vi "氨氮总磷质控流程.vi"(0 "队列输入":refnum<queue>, 5 "氨氮":bool, 7 "氨氮量程切换":enum32{"H", "L", "AUTO"}(ring)=enum."AUTO", 9 "总磷":bool, 11 "总磷量程切换":enum32{"H", "L", "AUTO"}(ring)=enum."AUTO") -> (4 "布尔":bool, 6 "总磷中断报警":bool, 8 "氨氮中断报警":bool)   [LabVIEW 2016, in "质控单元.lvlib"]
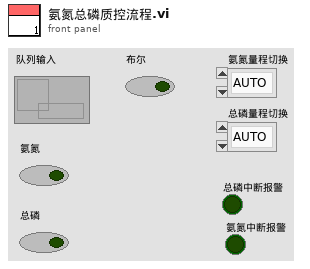
[diagram p1: front panel]
types:
  T1 = enum16{"待机", "启动氨氮水样", "氨氮测量中", "启动氨氮加标", "启动氨氮加标回收", "氨氮加标回收测量中", "启动总磷水样", "总磷水样测量中", "启动总磷加标", "启动总磷加标回收", "总磷加标回收测量中", "结束"}
  T2 = cluster{"站号":u16, "量程切换":enum32{"H", "L", "AUTO"}, "控制命令":enum16{"启动测量", "标样核查", "零点核查", "跨度核查", "空白测试", "平行样测试", "加标回收", "空白校准", "标样校准", "初始化（清洗）", "停止测试", "仪器重启", "校时", "模式设置", "测量间隔设置", "盲样测试"}, "模式设置":enum16{"待机", "连续模式", "周期模式", "定点模式", "受控模式", "手动模式"}, "测量间隔":u16}
  T3 = cluster{"时间标识":timestamp, "设备":string, "日志信息":string}
  T4 = cluster{"系统时间":timestamp, "工作状态":enum16{"空闲", "水样测试", "标样核查", "零点核查", "跨度核查", "空白测试", "平行样测试", "加标回收", "空白校准", "标样校准", "初始化（清洗）"}, "测量模式":enum16{"待机", "连续模式", "周期模式", "定点模式", "受控模式", "手动模式"}, "告警代码":enum16{"无告警", "缺试剂告警", "缺水样告警", "缺蒸馏水告警", "缺标液告警", "仪表漏液告警", "标定异常告警", "超量程告警", "加热异常", "低试剂预警", "超上限告警", "超下限告警", "仪表内部其他异常", "滴定异常告警", "电极异常告警", "量程切换告警", "参数设置告警", "PH电极电位异常", "电导率电极异常", "浊度光度异常", "溶解氧电极异常", "溶解氧光强异常", "温度异常告警", "PH异常告警", "溶解氧异常告警", "电导率异常告警", "浊度异常告警", "叶绿素异常告警", "藻密度异常告警", "蓝绿藻异常告警", "ORP异常告警", "氨氮异常告警", "清洁刷异常告警", "SD卡异常告警", "蓝牙异常告警", "Wifi异常告警", "流程异常告警"}, "故障代码":enum16{"无故障", "电机故障", "温度故障", "通讯故障", "滴定故障"}, "日志代码":u16, "软件版本":u16, "F0":sgl, "F1":sgl, "F2":sgl, "F3":sgl, "T":sgl, "H":sgl, "id":u16, "flowid":u16, "量程":u16, "总磷控温温度1":sgl, "营养盐控温温度2":sgl, "ADC":sgl}
  T5 = enum16{"空闲", "水样测试", "标样核查", "零点核查", "跨度核查", "空白测试", "平行样测试", "加标回收", "空白校准", "标样校准", "初始化（清洗）"}
  T6 = cluster{"因子编码":u32, "单位":u16, "标样参考值":sgl, "水样数据时间":timestamp, "水样实测值":sgl, "水样数据标识":string, "标样数据时间":timestamp, "标样实测值":sgl, "标样数据标识":string, "空白数据时间":timestamp, "空白实测值":sgl, "空白数据标识":string, "零点核查数据时间":timestamp, "零点核查实测值":sgl, "零点核查数据标识":string, "跨度核查数据时间":timestamp, "跨度核查实测值":sgl, "跨度核查数据标识":string, "加标回收数据时间":timestamp, "加标回收实测值":sgl, "加标回收数据标识":string, "平行样数据时间":timestamp, "平行样实测值":sgl, "平行样数据标识":string}
  T7 = cluster{"量程":dbl, "检出限":dbl, "加标前水样浓度":dbl, "加标后水样浓度":dbl, "加标水杯定容体积":dbl, "加标母液浓度":dbl, "加标体积":dbl, "加标回收率":dbl}
  T8 = cluster{"氨氮":u8, "总磷":u8, "总氮":u8, "CODMn":u8, "CODCr":u8}
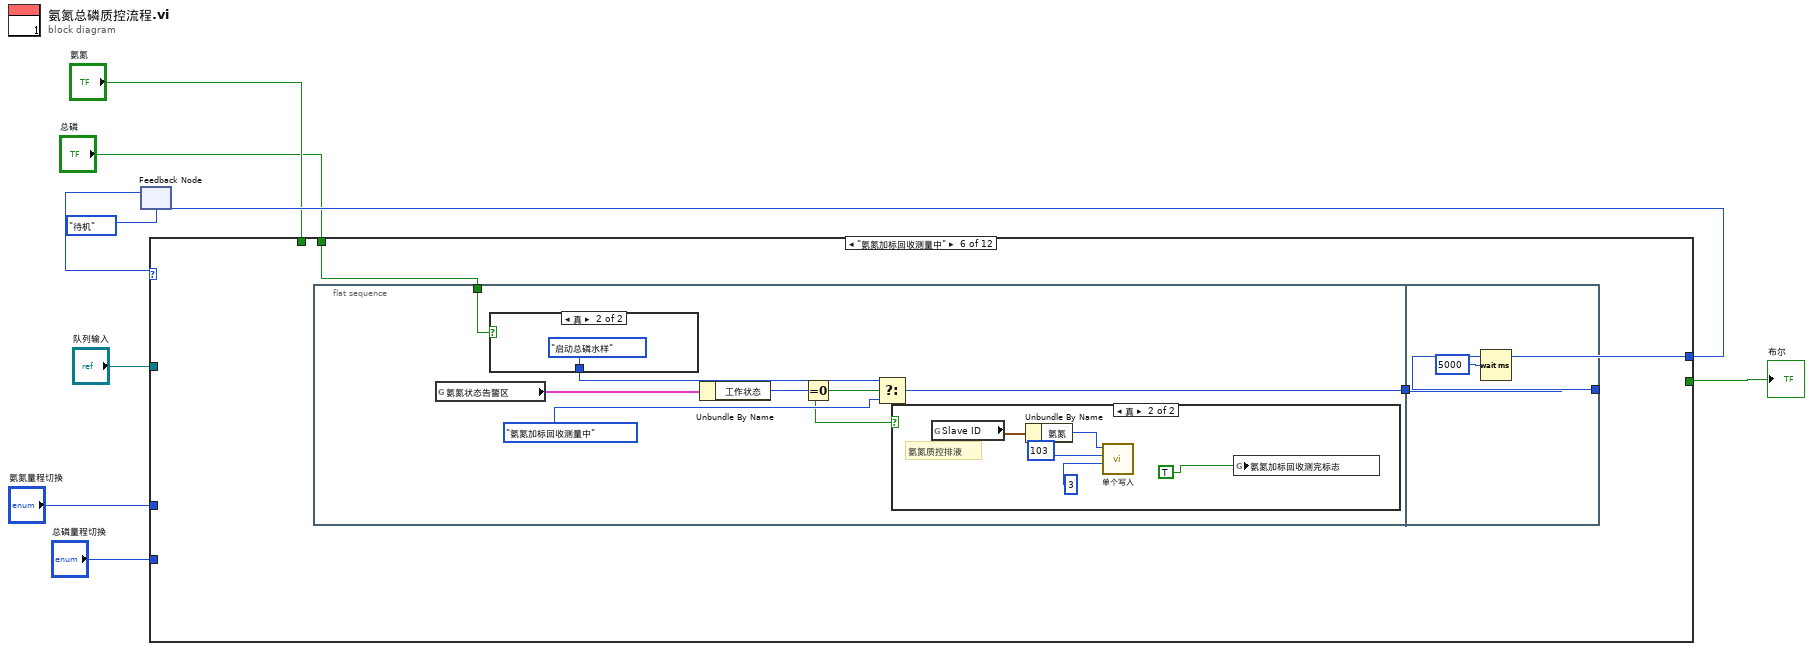
[diagram p0: block diagram]
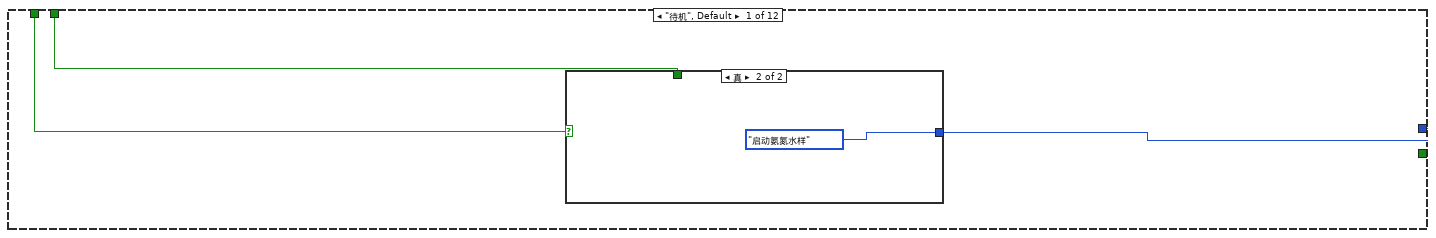
[diagram p2: hidden frame]
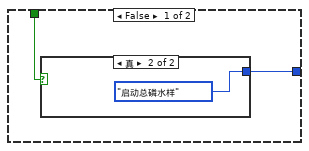
[diagram p3: hidden frame]
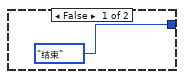
[diagram p4: hidden frame]
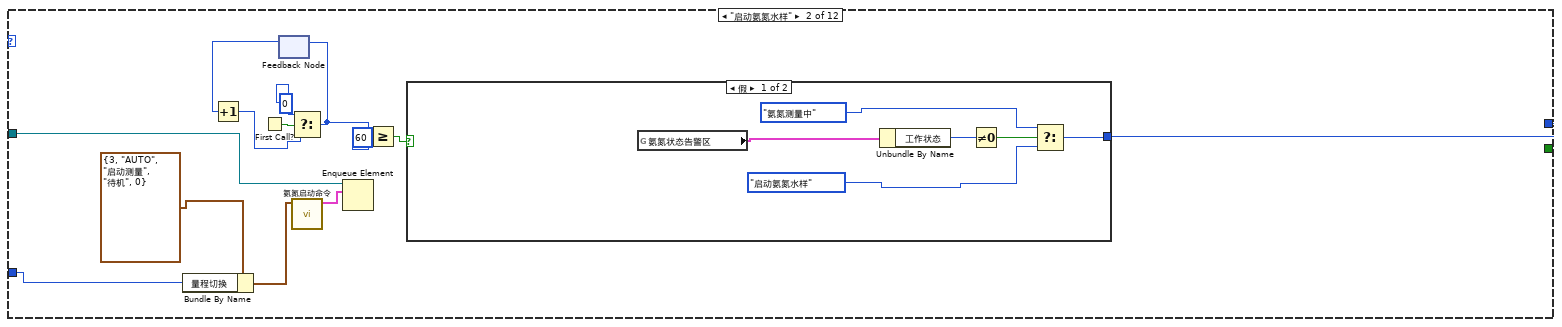
[diagram p5: hidden frame]
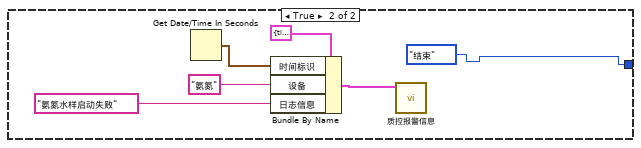
[diagram p6: hidden frame]
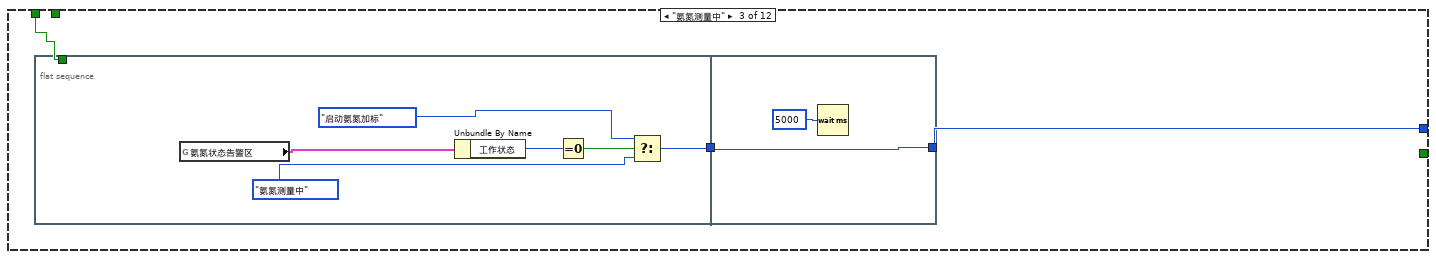
[diagram p7: hidden frame]
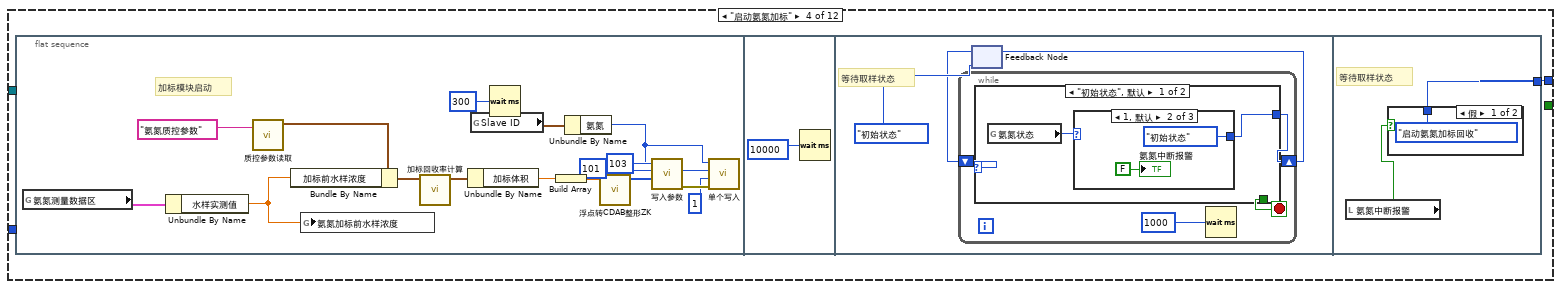
[diagram p8: hidden frame]
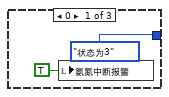
[diagram p9: hidden frame]
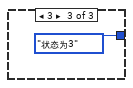
[diagram p10: hidden frame]
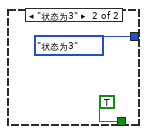
[diagram p11: hidden frame]
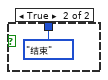
[diagram p12: hidden frame]
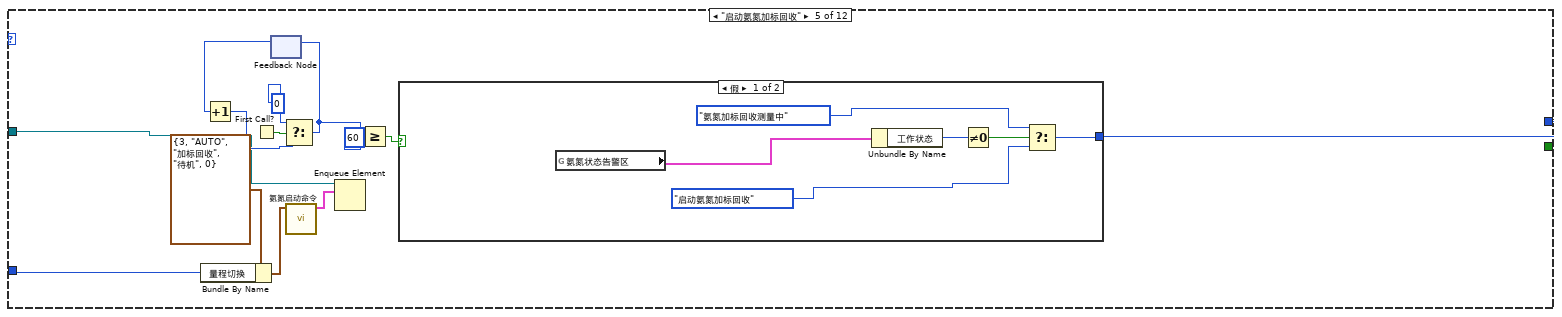
[diagram p13: hidden frame]
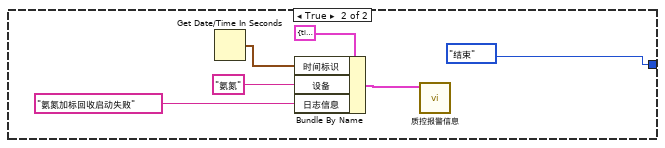
[diagram p14: hidden frame]
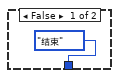
[diagram p15: hidden frame]
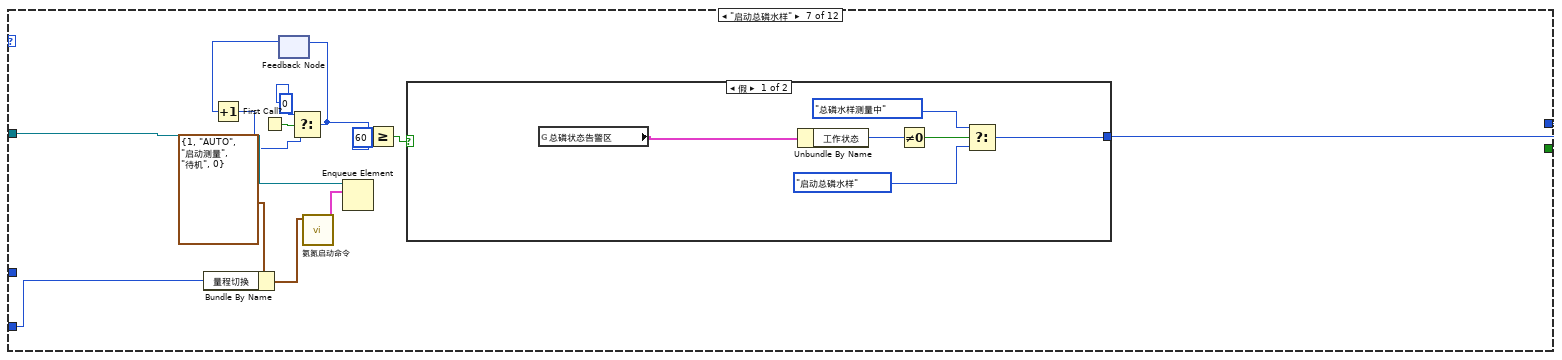
[diagram p17: hidden frame]
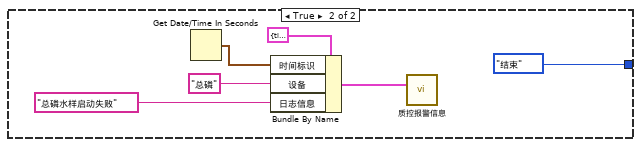
[diagram p18: hidden frame]
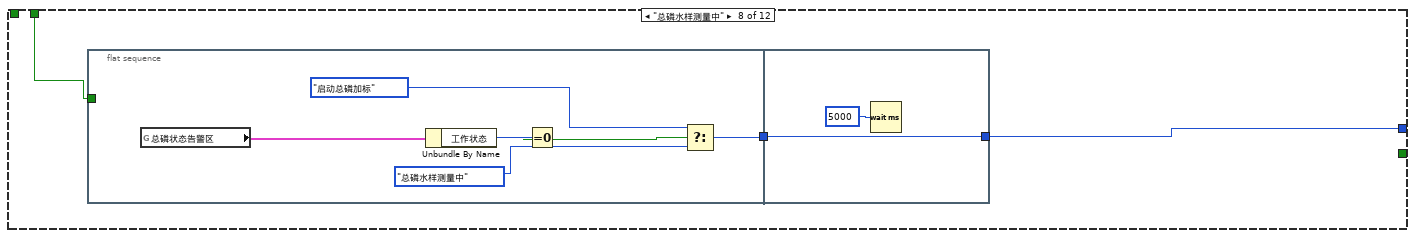
[diagram p19: hidden frame]
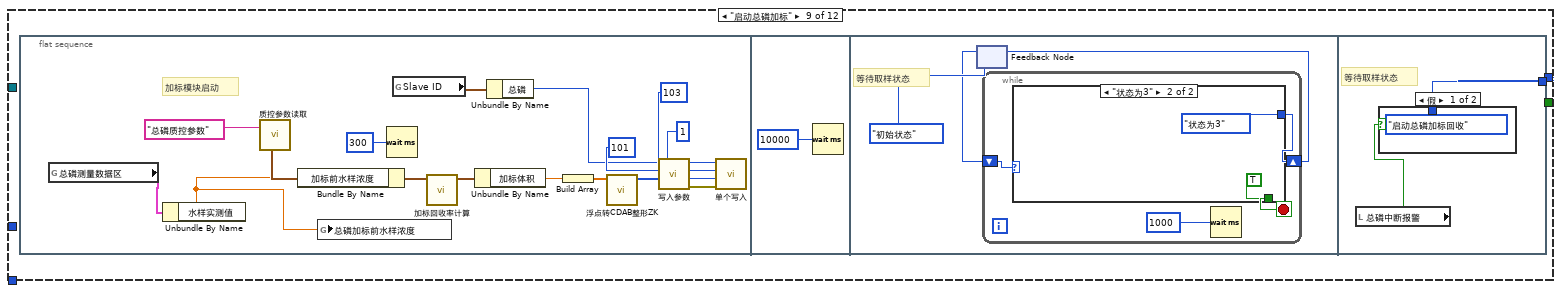
[diagram p20: hidden frame]
diagram:
  n1 = feedback #1(T1."待机") -> (w8:T1)
  n2 = case shown="\"氨氮加标回收测量中\"" w8 {
    tunnel: [w12 w29 w45 w54 w96 w118 w147 w163 w172 w214 w235 T1."结束"] -> w7
    tunnel: "队列输入" -> [_ w30 _ _ w97 _ w148 _ _ w215 _ _]
    tunnel: [_ _ _ _ _ _ _ _ _ _ _ TRUE] -> w4
    tunnel: "总磷" -> [w10 _ _ _ _ w117 _ w161 _ _ _ _]
    tunnel: "氨氮" -> [w11 _ w43 _ _ _ _ _ _ _ _ _]
    tunnel: "氨氮量程切换" -> [_ w19 _ _ w93 _ _ _ _ _ _ _]
    tunnel: "总磷量程切换" -> [_ _ _ _ _ _ w136 _ _ w213 _ _]
    frame "待机", Default {
      n3 = case shown="真" w11 {
        tunnel: [w13 T1."启动氨氮水样"] -> w12
        tunnel: w10 -> [w14 _]
        frame False {
          n4 = case shown="真" w14 {
            tunnel: [T1."结束" T1."启动总磷水样"] -> w13
            frame False {
            }
            frame True {
            }
          }
        }
        frame True {
        }
      }
    }
    frame "启动氨氮水样" {
      n5 = Bundle By Name(cluster=T2 {"站号"=3, "量程切换"=enum."AUTO", "控制命令"=enum."启动测量", "模式设置"=enum."待机", "测量间隔"=0} ("参数"), "量程切换"=w19) -> (w18:T2)
      n6 = First Call?() -> (First Call?: T/F=w27:bool)
      n7 = feedback #2() -> (w26:i32)  [unwired: 1 in]
      n8 = Increment(x=w26) -> (x+1=w25:i32)
      n9 = Select(t=0, s=w27, f=w25) -> (s? t:f=w24:i32)
      n10 = feedback-in #2(w24) -> ()
      n11 = call "氨氮启动命令.vi"("参数"=w18) -> ("启动命令"=w21:cluster{"命令":string, "data":variant})  [unwired: 10 in]
      n12 = Enqueue Element(queue=w30, element=w21) -> ()  [unwired: 2 in, 3 out]
      n13 = Greater Or Equal?(x=w24, y=60) -> (x >= y?=w22:bool)
      n14 = case shown="假" w22 {
        tunnel: [w34 T1."结束"] -> w29
        frame False {
          n15 = global read "与氨氮交互全局.vi" "氨氮状态告警区"() -> (w31:T4)
          n16 = Unbundle By Name(w31) -> ("工作状态"=w36:T5)
          n17 = Not Equal To 0?(x=w36) -> (x != 0?=w35:bool)
          n18 = Select(t=T1."氨氮测量中", s=w35, f=T1."启动氨氮水样") -> (s? t:f=w34:T1)
        }
        frame True {
          n19 = Get Date/Time In Seconds() -> (seconds since 1Jan1904=w42:timestamp)
          n20 = Bundle By Name(cluster=T3 {"时间标识"=timestamp(0 s since 1904-01-01), "设备"="", "日志信息"=""} ("data in"), "时间标识"=w42, "设备"="氨氮", "日志信息"="氨氮水样启动失败") -> (w38:T3)
          n21 = call "质控报警信息.vi"("data in"=w38) -> ()  [unwired: 11 in]
        }
      }
    }
    frame "氨氮测量中" {
      n22 = flat-sequence {
        tunnel: [w50] -> w44
        tunnel: w43 -> [_]
        tunnel: [w53] -> w45
        tunnel: w44 -> [w53]
        frame #0 {
          n23 = global read "与氨氮交互全局.vi" "氨氮状态告警区"() -> (w46:T4)
          n24 = Unbundle By Name(w46) -> ("工作状态"=w51:T5)
          n25 = Equal To 0?(x=w51) -> (x = 0?=w49:bool)
          n26 = Select(t=T1."启动氨氮加标", s=w49, f=T1."氨氮测量中") -> (s? t:f=w50:T1)
        }
        frame #1 {
          n27 = Wait (ms)(milliseconds to wait=u32 5000 ("等待时间（毫秒）")) -> ()  [unwired: 1 out]
        }
      }
    }
    frame "启动氨氮加标" {
      n28 = flat-sequence {
        tunnel: [w89] -> w54
        frame #0 {
          # "加标模块启动"
          n29 = global read "与氨氮交互全局.vi" "氨氮测量数据区"() -> (w58:T6)
          n30 = Unbundle By Name(w58) -> ("水样实测值"=w59:sgl)
          n31 = call "质控参数读取.vi"("section"="氨氮质控参数") -> ("参数"=w68:T7)  [unwired: 9 in, 1 out]
          n32 = Bundle By Name(cluster=w68, "加标前水样浓度"=w59) -> (w69:T7)
          n33 = global write "水样浓度全局.vi" "氨氮加标前水样浓度"(w59) -> ()
          n34 = call "加标回收率计算.vi"("参数"=w69) -> ("参数 out"=w67:T7)  [unwired: 9 in, 1 out]
          n35 = Unbundle By Name(w67) -> ("加标体积"=w60:dbl)
          n36 = global read "断电保存全局.vi" "Slave ID"() -> (w56:T8)
          n37 = Wait (ms)(milliseconds to wait=u32 300 ("等待时间（毫秒）")) -> ()  [unwired: 1 out]
          n38 = Build Array(w60) -> (w66:dbl[])
          n39 = Unbundle By Name(w56) -> ("氨氮"=w55:u8)
          n40 = call "浮点转CDAB整形ZK.vi"("浮点数"=w66) -> ("CDAB整形输出"=w61:u16[])  [unwired: 10 in]
          n41 = call "写入参数.vi"("values"=w61, "starting address"=u16 101, "Slave ID"=w55) -> ("error out"=w65:errorcluster)  [unwired: 8 in]
          n42 = call "单个写入.vi"("Error in"=w65, "value"=u16 1, "address"=u16 103, "Slave ID"=w55) -> ()  [unwired: 7 in, 1 out]
        }
        frame #1 {
          n43 = Wait (ms)(milliseconds to wait=u32 10000 ("等待时间（毫秒）")) -> ()  [unwired: 1 out]
        }
        frame #2 {
          # "等待取样状态"
          n44 = feedback #3(enum16{"初始状态", "状态为3"}."初始状态") -> (w73:enum16{"初始状态", "状态为3"})
          n45 = while {
            shift-right: [w77] -> w72
            shift-left: w73 -> [w78]
            stop <- w76 stop-if-true
            n46 = case shown="\"初始状态\", 默认" w78 {
              tunnel: [w80 enum16{"初始状态", "状态为3"}."状态为3"] -> w77
              tunnel: [_ TRUE] -> w76
              frame "初始状态", Default {
                n47 = global read "加标回收状态全局变量.vi" "氨氮状态"() -> (w79:u16)
                n48 = case shown="1, 默认" w79 {
                  tunnel: [enum16{"初始状态", "状态为3"}."状态为3" enum16{"初始状态", "状态为3"}."初始状态" enum16{"初始状态", "状态为3"}."状态为3"] -> w80
                  frame 0 {
                    n49 = local write "氨氮中断报警"(TRUE ("氨氮中断报警")) -> ()
                  }
                  frame 1, Default {
                    "氨氮中断报警" <- FALSE ("氨氮中断报警")
                  }
                  frame 3 {
                  }
                }
              }
              frame "状态为3" {
              }
            }
            n50 = Wait (ms)(milliseconds to wait=u32 1000 ("等待时间（毫秒）")) -> ()  [unwired: 1 out]
          }
          n51 = feedback-in #3(w72) -> ()
        }
        frame #3 {
          # "等待取样状态"
          n52 = local read "氨氮中断报警"() -> (w88:bool)
          n53 = case shown="假" w88 {
            tunnel: [T1."启动氨氮加标回收" T1."结束"] -> w89
            frame False {
            }
            frame True {
            }
          }
        }
      }
    }
    frame "启动氨氮加标回收" {
      n54 = Bundle By Name(cluster=T2 {"站号"=3, "量程切换"=enum."AUTO", "控制命令"=enum."加标回收", "模式设置"=enum."待机", "测量间隔"=0} ("参数"), "量程切换"=w93) -> (w92:T2)
      n55 = First Call?() -> (First Call?: T/F=w103:bool)
      n56 = feedback #4() -> (w102:i32)  [unwired: 1 in]
      n57 = Increment(x=w102) -> (x+1=w101:i32)
      n58 = Select(t=0, s=w103, f=w101) -> (s? t:f=w100:i32)
      n59 = feedback-in #4(w100) -> ()
      n60 = call "氨氮启动命令.vi"("参数"=w92) -> ("启动命令"=w95:cluster{"命令":string, "data":variant})  [unwired: 10 in]
      n61 = Enqueue Element(queue=w97, element=w95) -> ()  [unwired: 2 in, 3 out]
      n62 = Greater Or Equal?(x=w100, y=60) -> (x >= y?=w98:bool)
      n63 = case shown="假" w98 {
        tunnel: [w108 T1."结束"] -> w96
        frame False {
          n64 = global read "与氨氮交互全局.vi" "氨氮状态告警区"() -> (w105:T4)
          n65 = Unbundle By Name(w105) -> ("工作状态"=w110:T5)
          n66 = Not Equal To 0?(x=w110) -> (x != 0?=w109:bool)
          n67 = Select(t=T1."氨氮加标回收测量中", s=w109, f=T1."启动氨氮加标回收") -> (s? t:f=w108:T1)
        }
        frame True {
          n68 = Get Date/Time In Seconds() -> (seconds since 1Jan1904=w116:timestamp)
          n69 = Bundle By Name(cluster=T3 {"时间标识"=timestamp(0 s since 1904-01-01), "设备"="", "日志信息"=""} ("data in"), "时间标识"=w116, "设备"="氨氮", "日志信息"="氨氮加标回收启动失败") -> (w112:T3)
          n70 = call "质控报警信息.vi"("data in"=w112) -> ()  [unwired: 11 in]
        }
      }
    }
    frame "氨氮加标回收测量中" {
      n71 = flat-sequence {
        tunnel: [w125] -> w119
        tunnel: w117 -> [w121]
        tunnel: [w135] -> w118
        tunnel: w119 -> [w135]
        frame #0 {
          n72 = global read "与氨氮交互全局.vi" "氨氮状态告警区"() -> (w120:T4)
          n73 = case shown="真" w121 {
            tunnel: [T1."结束" T1."启动总磷水样"] -> w123
            frame False {
            }
            frame True {
            }
          }
          n74 = Unbundle By Name(w120) -> ("工作状态"=w126:T5)
          n75 = Equal To 0?(x=w126) -> (x = 0?=w122:bool)
          n76 = Select(t=w123, s=w122, f=T1."氨氮加标回收测量中") -> (s? t:f=w125:T1)
          n77 = case shown="真" w122 {
            frame False {
            }
            frame True {
              # "氨氮质控排液"
              n78 = global read "断电保存全局.vi" "Slave ID"() -> (w130:T8)
              n79 = Unbundle By Name(w130) -> ("氨氮"=w129:u8)
              n80 = call "单个写入.vi"("value"=u16 3, "address"=u16 103, "Slave ID"=w129) -> ()  [unwired: 8 in, 1 out]
              n81 = global write "质控测完标志全局 1.vi" "氨氮加标回收测完标志"(TRUE) -> ()
            }
          }
        }
        frame #1 {
          n82 = Wait (ms)(milliseconds to wait=u32 5000 ("等待时间（毫秒）")) -> ()  [unwired: 1 out]
        }
      }
    }
    frame "启动总磷水样" {
      n83 = Bundle By Name(cluster=T2 {"站号"=1, "量程切换"=enum."AUTO", "控制命令"=enum."启动测量", "模式设置"=enum."待机", "测量间隔"=0} ("参数"), "量程切换"=w136) -> (w138:T2)
      n84 = First Call?() -> (First Call?: T/F=w145:bool)
      n85 = feedback #5() -> (w144:i32)  [unwired: 1 in]
      n86 = Increment(x=w144) -> (x+1=w143:i32)
      n87 = Select(t=0, s=w145, f=w143) -> (s? t:f=w142:i32)
      n88 = feedback-in #5(w142) -> ()
      n89 = call "氨氮启动命令.vi"("参数"=w138) -> ("启动命令"=w137:cluster{"命令":string, "data":variant})  [unwired: 10 in]
      n90 = Enqueue Element(queue=w148, element=w137) -> ()  [unwired: 2 in, 3 out]
      n91 = Greater Or Equal?(x=w142, y=60) -> (x >= y?=w140:bool)
      n92 = case shown="假" w140 {
        tunnel: [w152 T1."结束"] -> w147
        frame False {
          n93 = global read "与总磷交互全局.vi" "总磷状态告警区"() -> (w149:T4)
          n94 = Unbundle By Name(w149) -> ("工作状态"=w153:T5)
          n95 = Not Equal To 0?(x=w153) -> (x != 0?=w154:bool)
          n96 = Select(t=T1."总磷水样测量中", s=w154, f=T1."启动总磷水样") -> (s? t:f=w152:T1)
        }
        frame True {
          n97 = Get Date/Time In Seconds() -> (seconds since 1Jan1904=w160:timestamp)
          n98 = Bundle By Name(cluster=T3 {"时间标识"=timestamp(0 s since 1904-01-01), "设备"="", "日志信息"=""} ("data in"), "时间标识"=w160, "设备"="总磷", "日志信息"="总磷水样启动失败") -> (w156:T3)
          n99 = call "质控报警信息.vi"("data in"=w156) -> ()  [unwired: 11 in]
        }
      }
    }
    frame "总磷水样测量中" {
      n100 = flat-sequence {
        tunnel: [w168] -> w162
        tunnel: w161 -> [_]
        tunnel: [w171] -> w163
        tunnel: w162 -> [w171]
        frame #0 {
          n101 = global read "与总磷交互全局.vi" "总磷状态告警区"() -> (w164:T4)
          n102 = Unbundle By Name(w164) -> ("工作状态"=w169:T5)
          n103 = Equal To 0?(x=w169) -> (x = 0?=w167:bool)
          n104 = Select(t=T1."启动总磷加标", s=w167, f=T1."总磷水样测量中") -> (s? t:f=w168:T1)
        }
        frame #1 {
          n105 = Wait (ms)(milliseconds to wait=u32 5000 ("等待时间（毫秒）")) -> ()  [unwired: 1 out]
        }
      }
    }
    frame "启动总磷加标" {
      n106 = flat-sequence {
        tunnel: [w207] -> w172
        frame #0 {
          # "加标模块启动"
          n107 = global read "与总磷交互全局.vi" "总磷测量数据区"() -> (w175:T6)
          n108 = Unbundle By Name(w175) -> ("水样实测值"=w177:sgl)
          n109 = call "质控参数读取.vi"("section"="总磷质控参数") -> ("参数"=w178:T7)  [unwired: 9 in, 1 out]
          n110 = Bundle By Name(cluster=w178, "加标前水样浓度"=w177) -> (w187:T7)
          n111 = global write "水样浓度全局.vi" "总磷加标前水样浓度"(w177) -> ()
          n112 = Wait (ms)(milliseconds to wait=u32 300 ("等待时间（毫秒）")) -> ()  [unwired: 1 out]
          n113 = global read "断电保存全局.vi" "Slave ID"() -> (w174:T8)
          n114 = call "加标回收率计算.vi"("参数"=w187) -> ("参数 out"=w186:T7)  [unwired: 9 in, 1 out]
          n115 = Unbundle By Name(w186) -> ("加标体积"=w179:dbl)
          n116 = Unbundle By Name(w174) -> ("总磷"=w173:u8)
          n117 = Build Array(w179) -> (w185:dbl[])
          n118 = call "浮点转CDAB整形ZK.vi"("浮点数"=w185) -> ("CDAB整形输出"=w180:u16[])  [unwired: 10 in]
          n119 = call "写入参数.vi"("values"=w180, "starting address"=u16 101, "Slave ID"=w173) -> ("error out"=w184:errorcluster)  [unwired: 8 in]
          n120 = call "单个写入.vi"("Error in"=w184, "value"=u16 1, "address"=u16 103, "Slave ID"=w173) -> ()  [unwired: 7 in, 1 out]
        }
        frame #1 {
          n121 = Wait (ms)(milliseconds to wait=u32 10000 ("等待时间（毫秒）")) -> ()  [unwired: 1 out]
        }
        frame #2 {
          # "等待取样状态"
          n122 = feedback #6(enum16{"初始状态", "状态为3"}."初始状态") -> (w191:enum16{"初始状态", "状态为3"})
          n123 = while {
            shift-right: [w195] -> w190
            shift-left: w191 -> [w196]
            stop <- w194 stop-if-true
            n124 = case shown="\"状态为3\"" w196 {
              tunnel: [w198 enum16{"初始状态", "状态为3"}."状态为3"] -> w195
              tunnel: [_ TRUE] -> w194
              frame "初始状态", Default {
                n125 = global read "加标回收状态全局变量.vi" "总磷状态"() -> (w197:u16)
                n126 = case shown="3" w197 {
                  tunnel: [enum16{"初始状态", "状态为3"}."状态为3" enum16{"初始状态", "状态为3"}."初始状态" enum16{"初始状态", "状态为3"}."状态为3"] -> w198
                  frame 0 {
                    n127 = local write "总磷中断报警"(TRUE ("总磷中断报警")) -> ()
                  }
                  frame 1, Default {
                    "总磷中断报警" <- FALSE ("总磷中断报警")
                  }
                  frame 3 {
                  }
                }
              }
              frame "状态为3" {
              }
            }
            n128 = Wait (ms)(milliseconds to wait=u32 1000 ("等待时间（毫秒）")) -> ()  [unwired: 1 out]
          }
          n129 = feedback-in #6(w190) -> ()
        }
        frame #3 {
          # "等待取样状态"
          n130 = local read "总磷中断报警"() -> (w206:bool)
          n131 = case shown="假" w206 {
            tunnel: [T1."启动总磷加标回收" T1."结束"] -> w207
            frame False {
            }
            frame True {
            }
          }
        }
      }
    }
    frame "启动总磷加标回收" {
      n132 = Bundle By Name(cluster=T2 {"站号"=1, "量程切换"=enum."AUTO", "控制命令"=enum."加标回收", "模式设置"=enum."待机", "测量间隔"=0} ("参数"), "量程切换"=w213) -> (w211:T2)
      n133 = First Call?() -> (First Call?: T/F=w221:bool)
      n134 = feedback #7() -> (w220:i32)  [unwired: 1 in]
      n135 = Increment(x=w220) -> (x+1=w219:i32)
      n136 = Select(t=0, s=w221, f=w219) -> (s? t:f=w218:i32)
      n137 = feedback-in #7(w218) -> ()
      n138 = call "氨氮启动命令.vi"("参数"=w211) -> ("启动命令"=w210:cluster{"命令":string, "data":variant})  [unwired: 10 in]
      n139 = Enqueue Element(queue=w215, element=w210) -> ()  [unwired: 2 in, 3 out]
      n140 = Greater Or Equal?(x=w218, y=60) -> (x >= y?=w216:bool)
      n141 = case shown="假" w216 {
        tunnel: [w227 T1."结束"] -> w214
        frame False {
          n142 = global read "与总磷交互全局.vi" "总磷状态告警区"() -> (w224:T4)
          n143 = Unbundle By Name(w224) -> ("工作状态"=w223:T5)
          n144 = Not Equal To 0?(x=w223) -> (x != 0?=w228:bool)
          n145 = Select(t=T1."总磷加标回收测量中", s=w228, f=T1."启动总磷加标回收") -> (s? t:f=w227:T1)
        }
        frame True {
          n146 = Get Date/Time In Seconds() -> (seconds since 1Jan1904=w234:timestamp)
          n147 = Bundle By Name(cluster=T3 {"时间标识"=timestamp(0 s since 1904-01-01), "设备"="", "日志信息"=""} ("data in"), "时间标识"=w234, "设备"="总磷", "日志信息"="总磷启动失败") -> (w230:T3)
          n148 = call "质控报警信息.vi"("data in"=w230) -> ()  [unwired: 11 in]
        }
      }
    }
    frame "总磷加标回收测量中" {
      n149 = flat-sequence {
        tunnel: [w242] -> w236
        tunnel: [w249] -> w235
        tunnel: w236 -> [w249]
        frame #0 {
          n150 = global read "与总磷交互全局.vi" "总磷状态告警区"() -> (w238:T4)
          n151 = Unbundle By Name(w238) -> ("工作状态"=w237:T5)
          n152 = Equal To 0?(x=w237) -> (x = 0?=w239:bool)
          n153 = Select(t=T1."结束", s=w239, f=T1."总磷加标回收测量中") -> (s? t:f=w242:T1)
          n154 = case shown="真" w239 {
            frame False {
            }
            frame True {
              # "总磷质控排液"
              n155 = global read "断电保存全局.vi" "Slave ID"() -> (w244:T8)
              n156 = global write "质控测完标志全局 1.vi" "总磷加标回收测完标志"(TRUE) -> ()
              n157 = Unbundle By Name(w244) -> ("总磷"=w243:u8)
              n158 = call "单个写入.vi"("value"=u16 3, "address"=u16 103, "Slave ID"=w243) -> ()  [unwired: 8 in, 1 out]
            }
          }
        }
        frame #1 {
          n159 = Wait (ms)(milliseconds to wait=u32 5000 ("等待时间（毫秒）")) -> ()  [unwired: 1 out]
        }
      }
    }
    frame "结束" {
    }
  }
  "布尔" <- w4
  n160 = feedback-in #1(w7) -> ()
